vi "ConvertActiveChannelSelectionsToBinary.vi"(8 "error in (no error)":errorcluster, 11 "Active Channels":T1) -> (0 "error out":errorcluster, 3 "Active Channels":i32)   [LabVIEW 2023, in "Thermotron 8800.lvlib"]
uses:
  Thermotron 8800.lvlib
  ActiveChannels.ctl
panel:
  out "binary string":string
  out "Active Channels binary":i32
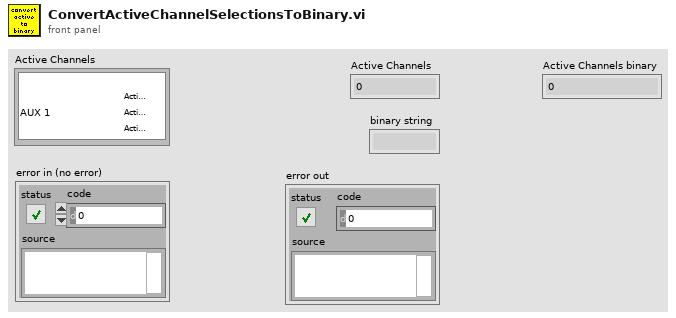
[diagram p1: front panel]
types:
  T1 = typedef "Thermotron 8800.lvlib/ActiveChannels.ctl" = i32[]
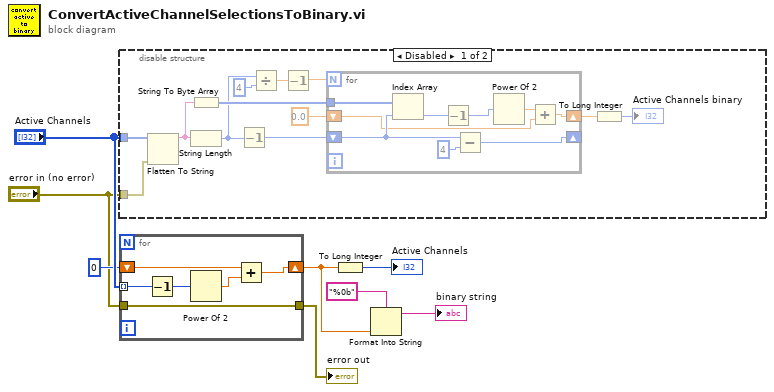
[diagram p0: block diagram]
diagram:
  n1 = disable-structure shown="Disabled" {
    disable-tunnel: "Active Channels" -> [w10 _]
    disable-tunnel: "error in (no error)" -> [w9 _]
    frame Disabled {
      n2 = Flatten To String(anything=w10, error in (no error)=w9) -> (data string=w12:string)  [unwired: 2 in, 2 out]
      n3 = String To Byte Array(string=w12) -> (unsigned byte array=w17:u8[])
      n4 = String Length(string=w12) -> (length=w16:i32)
      n5 = Decrement(x=w16) -> (x-1=w18:i32)
      n6 = Divide(x=w16, y=4) -> (x/y=w14:dbl)
      n7 = Decrement(x=w14) -> (x-1=w15:dbl)
      n8 = for {
        N: w15 -> [_]
        tunnel: w17 -> [w29]
        shift-right: [w26] -> _
        shift-left: w18 -> [w28]
        shift-right: [w21] -> w20
        shift-left: 0.0 -> [w22]
        n9 = Index Array(array=w29, index=w28) -> (element=w25:u8)
        n10 = Decrement(x=w25) -> (x-1=w24:u8)
        n11 = Subtract(x=w28, y=4) -> (x-y=w26:i32)
        n12 = Power Of 2(x=w24) -> (2^x=w23:dbl)
        n13 = Add(x=w23, y=w22) -> (x+y=w21:dbl)
      }
      n14 = To Long Integer(number=w20) -> (32bit integer=→"Active Channels binary":i32)
    }
    frame Enabled {
    }
  }
  n15 = for {
    tunnel: "Active Channels" -> [w33] mode=indexing
    shift-right: [w34] -> w4
    shift-left: 0 -> [w35]
    tunnel: "error in (no error)" -> [w30]
    tunnel: [w30] -> w1
    n16 = Decrement(x=w33) -> (x-1=w32:i32)
    n17 = Power Of 2(x=w32) -> (2^x=w31:dbl)
    n18 = Add(x=w35, y=w31) -> (x+y=w34:dbl)
  }
  "error out" <- w1
  n19 = To Long Integer(number=w4) -> (32bit integer=→"Active Channels":i32)
  n20 = Format Into String(format string="%0b", w4) -> (resulting string=→"binary string":string)  [unwired: 2 in, 1 out]
